vi "Read Voltage Setpoint (Single).vi"(8 "error in":errorcluster, 9 "Channel Index":i32=1, 11 "Voltage Control in":refnum<class "Voltage Control.lvclass">) -> (0 "error out":errorcluster, 1 "Changed or First Call?":bool, 2 "Voltage Setpoint":dbl, 3 "Voltage Control out":refnum<class "Voltage Control.lvclass">)   [LabVIEW 2023, in "Voltage Control.lvclass"]
doc: "This VI will read a single Channel's setpoint. The <b>Channel Index</b> input is 1-based."
uses:
  Voltage Control.lvclass
  Voltage Control.lvclass/Voltage Control.ctl
  <vilib>/ADAS Replay HIL/Channels/Tag Wrapper/Polymorphic/Read Channel (Double).vi
  19ddb35d-a8bc-47ec-aa8f-2c2e4404ec76.vi
  <vilib>/ADAS Replay HIL/Channels/Tag Wrapper/Polymorphic/Read Channel (Double).vi/b2f764de-0c1e-4784-a155-687fc995a684.vi
  <vilib>/ADAS Replay HIL/Channels/Tag Wrapper/Polymorphic/Read Channel (Double).vi/b2f764de-0c1e-4784-a155-687fc995a684.vi/c28b0ead-42ad-4072-80a2-aca7f2bd7ce3.vi
  <vilib>/ADAS Replay HIL/Channels/Tag Wrapper/Polymorphic/Read Channel (Double).vi/b2f764de-0c1e-4784-a155-687fc995a684.vi/219d0231-d98b-4193-b5cc-84f90e3c9091.vi
  <vilib>/ADAS Replay HIL/Channels/Tag Wrapper/Tag Wrapper.lvlib
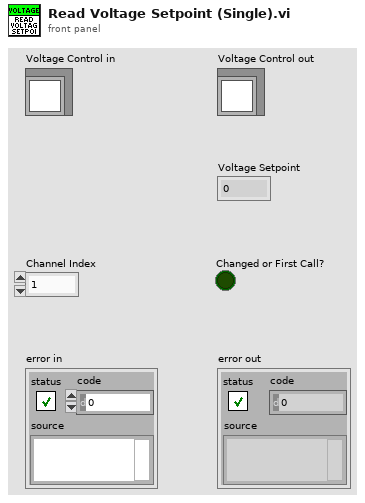
[diagram p1: front panel]
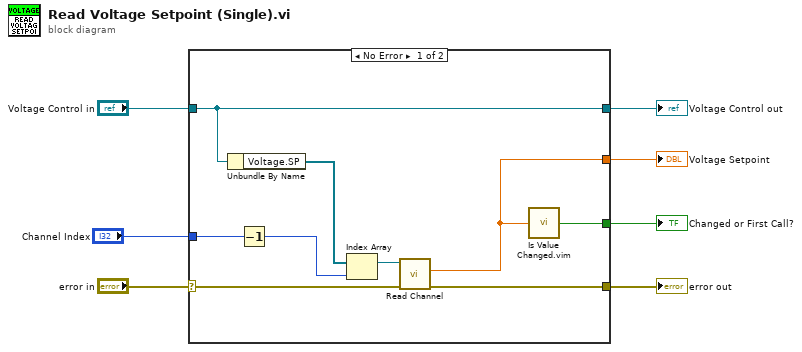
[diagram p0: block diagram]
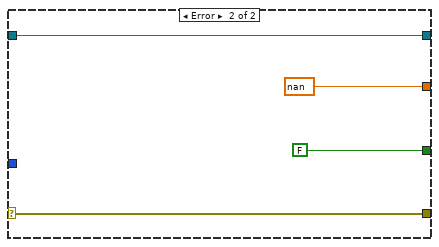
[diagram p2: hidden frame]
diagram:
  n1 = case shown="No Error" "error in" {
    selector: "error in" -> [w14 w20]
    tunnel: [w13 w20] -> w5
    tunnel: [w16 w19] -> w4
    tunnel: "Voltage Control in" -> [w16 w19]
    tunnel: [w12 nan ("Value out")] -> w7
    tunnel: [w11 FALSE ("changed or first call?")] -> w6
    tunnel: "Channel Index" -> [w9 _]
    frame No Error {
      n2 = Unbundle By Name(w16) -> ("Voltage.SP"=w15:refnum<k21>[])
      n3 = Decrement(x=w9) -> (x-1=w8:i32)
      n4 = Index Array(array=w15, index=w8) -> (element=w10:refnum<k21>)
      n5 = call-poly <vilib>:"Read Channel.vi"("error in"=w14, "ADAS HIL Channel in"=w10) -> ("error out"=w13:errorcluster, "Value out"=w12:dbl)  [unwired: 6 in, 2 out]
      n6 = call "Is Value Changed.vim"("value"=w12) -> ("changed or first call?"=w11:bool)
    }
    frame Error {
    }
  }
  "error out" <- w5
  "Voltage Control out" <- w4
  "Voltage Setpoint" <- w7
  "Changed or First Call?" <- w6
